vi "InverseKinematics.vi"(0 "Next X":dbl, 2 "deltaY":dbl, 3 "deltaX":dbl, 5 "Next Y":dbl, 7 "L0":dbl, 9 "L1":dbl, 11 "error in (no error)":errorcluster) -> (4 "destheta0":dbl, 6 "destheta1":dbl, 15 "error out":errorcluster)   [LabVIEW 2017, in "admittanceControllerLibrary.lvlib"]
doc: "This VI uses a mathscript node to perform the Inverse Kinematics, which turns the desired location into a desired joint angle (degrees)."
uses:
  admittanceControllerLibrary.lvlib
  <vilib>/imath/engines/lvmath2/RunTimeEngine/ArithmeticOperatorToken/NIMS_ArithmeticOperator_power(S).vi
  <instcachedir>/0/NIMS_ArithmeticOperator_power(S)_86B1D76B77564424912EAFCCCC7488ED.lvgen/NIMS_ArithmeticOperator_power(S)_86B1D76B77564424912EAFCCCC7488ED_010.vi
  <vilib>/imath/engines/lvmath2/RunTimeEngine/BuiltInFunctions/acos/NIMS_acos(C).vi
  <instcachedir>/0/NIMS_acos(C)_09AB0EA1D77D44F8AD620F57E6E2841E.lvgen/NIMS_acos(C)_09AB0EA1D77D44F8AD620F57E6E2841E_001.vi
  <vilib>/imathl/engines/lvmath/Functions/Error Handling/Create Error.vi
  <vilib>/imath/engines/lvmath2/RunTimeSupport/NIMS_Complex To Real.vi
  <instcachedir>/0/NIMS_Complex To Real_BE01396FDE034E8E94CEBBA1E368668D.lvgen/NIMS_Complex To Real_BE01396FDE034E8E94CEBBA1E368668D_001.vi
  <vilib>/imath/engines/lvmath2/RunTimeEngine/BuiltInFunctions/rad_to_deg/NIMS_rad_to_deg.vi
  <instcachedir>/0/NIMS_rad_to_deg_A39AFCDDC8C049FCADAAB7FC30B9F5AA.lvgen/NIMS_rad_to_deg_A39AFCDDC8C049FCADAAB7FC30B9F5AA_001.vi
  <vilib>/imath/engines/lvmath2/RunTimeEngine/NodeEndStatement/NIMS_NodeEndStatement_Output.vi
  <instcachedir>/0/NIMS_NodeEndStatement_Output_53EC0D466D134D7ABD903AC30B43404B.lvgen/NIMS_NodeEndStatement_Output_53EC0D466D134D7ABD903AC30B43404B_001.vi
  <vilib>/imath/engines/lvmath2/RunTimeEngine/ErrorHandling/NIMS_Finalize Error.vi
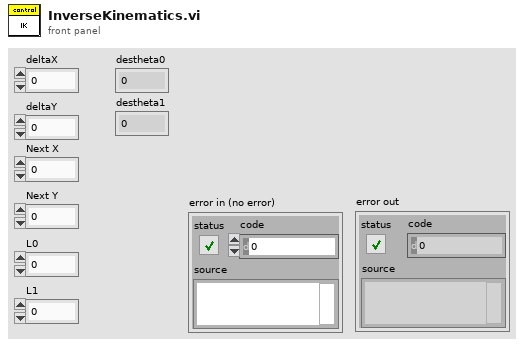
[diagram p1: front panel]
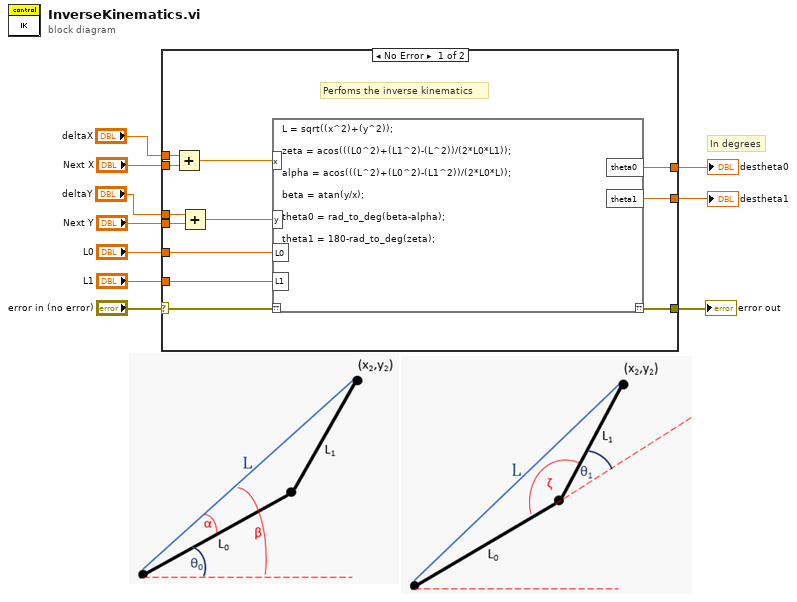
[diagram p0: block diagram]
diagram:
  # "In degrees"
  n1 = case shown="No Error" "error in (no error)" {
    selector: "error in (no error)" -> [w12 w166]
    tunnel: "L0" -> [w22 _]
    tunnel: "L1" -> [w21 _]
    tunnel: [w20 _] -> w8
    tunnel: [w19 _] -> w7
    tunnel: "deltaX" -> [w18 _]
    tunnel: "Next X" -> [w17 _]
    tunnel: "Next Y" -> [w15 _]
    tunnel: "deltaY" -> [w14 _]
    tunnel: [w11 w166] -> w1
    frame No Error {
      # "Perfoms the inverse kinematics"
      n2 = Add(x=w18, y=w17) -> (x+y=w16:dbl)
      n3 = Add(x=w14, y=w15) -> (x+y=w13:dbl)
      n4 = mathscript code="L = sqrt((x^2)+(y^2));\n\nzeta = acos(((L0^2)+(L1^2)-(L^2))/(2*L0*L1));\n\nalpha = acos(((L^2)+(L0^2)-(L1^2))/(2*L0*L));\n\nbeta = atan(y/x);\n\ntheta0 = rad_to_deg(beta-alpha);\n\ntheta1 = 180-rad_to_deg(zeta);"("??"=w12, "x"=w16, "y"=w13, "L0"=w22, "L1"=w21) -> ("??"=w11:errorcluster, "theta0"=w20:dbl, "theta1"=w19:dbl)
    }
    frame Error {
    }
  }
  "destheta0" <- w8
  "destheta1" <- w7
  "error out" <- w1
